vi "Open.vi"(8 "error in (no error)":errorcluster, 11 "MelsecTCP in":refnum<class "MelsecMcNet.lvclass">) -> (0 "error out":errorcluster, 3 "MelsecTCP out":refnum<class "MelsecMcNet.lvclass">)   [LabVIEW 2020, in "HslCommunication.lvlib" / "MelsecMcNet.lvclass"]
uses:
  MelsecMcNet.lvclass
  MelsecMcNet.lvclass/MelsecMcNet.ctl
  E:/Git/Libraries/develop/HslCommunication/_Dependenciecs/HslCommunication.dll
  _Dependenciecs/HslCommunication.dll
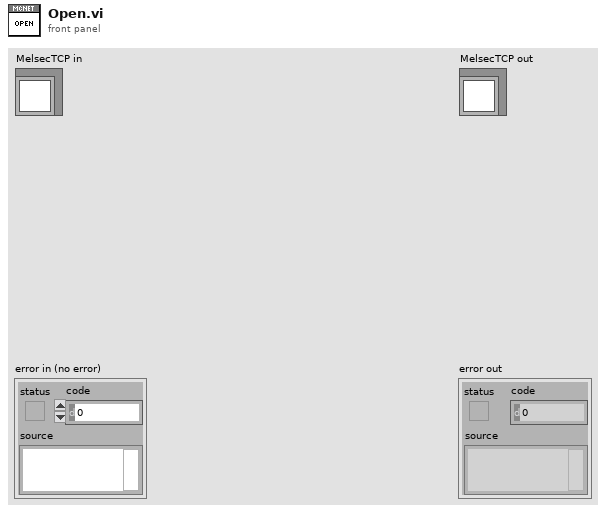
[diagram p1: front panel]
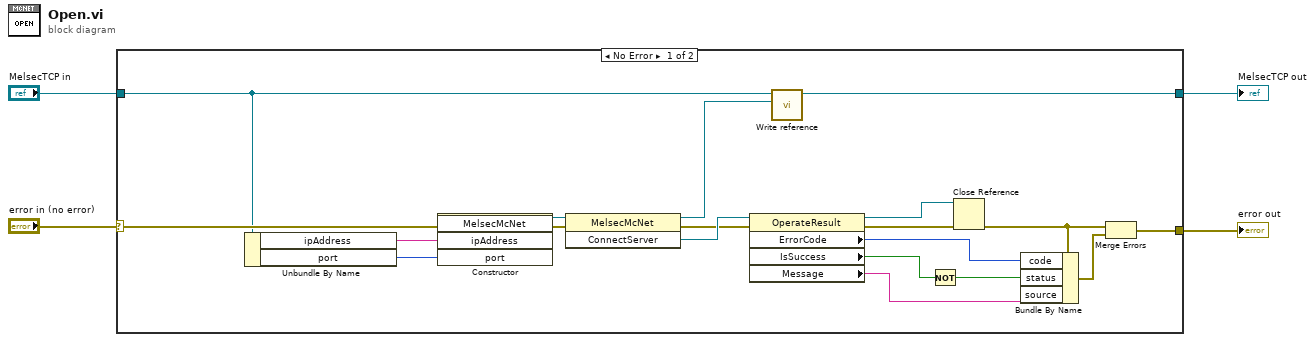
[diagram p0: block diagram]
diagram:
  n1 = case shown="No Error" "error in (no error)" {
    selector: "error in (no error)" -> [w8 w25]
    tunnel: "MelsecTCP in" -> [w6 w24]
    tunnel: [w5 w24] -> w1
    tunnel: [w19 w25] -> w2
    frame No Error {
      n2 = Unbundle By Name(w6) -> ("ipAddress"=w12:string, "port"=w11:i32)
      n3 = constructor class="MelsecMcNet"(error in=w8, "ipAddress"=w12, "port"=w11) -> (reference out=w10:refnum<k24>, error out=w9:errorcluster)  [unwired: 2 in, 3 out]
      n4 = invoke class="MelsecMcNet" method="ConnectServer"(reference=w10, error in=w9) -> (reference out=w7:refnum<k24>, error out=w14:errorcluster, "ConnectServer"=w15:refnum<k24>)  [unwired: 1 in]
      n5 = property class="OperateResult"(reference=w15, error in=w14) -> (reference out=w18:refnum<k24>, error out=w17:errorcluster, "ErrorCode"=w22:i32, "IsSuccess"=w16:bool, "Message"=w20:string)
      n6 = call-dynamic "Write reference.vi"("reference"=w7, "MelsecMcNet in"=w6) -> ("MelsecMcNet out"=w5:refnum<class "MelsecMcNet.lvclass">)  [unwired: 8 in, 1 out]
      n7 = Not(x=w16) -> (.not. x?=w21:bool)
      n8 = Close Reference(reference=w18, error in (no error)=w17) -> (error out=w13:errorcluster)
      n9 = Bundle By Name(cluster=w13, "code"=w22, "status"=w21, "source"=w20) -> (w23:errorcluster)
      n10 = Merge Errors(w13, w23) -> (w19:errorcluster)
    }
    frame Error {
    }
  }
  "error out" <- w2
  "MelsecTCP out" <- w1
